vi "GetSensorType(hackversion).vi"(11 "Accessors:ID":string) -> (2 "offset":i32, 3 "SensorType":T1 items=["BumperSensor"=1, "DistanceSensor"=2, "AccelerometerSensor"=3, "Wall Sensor"=4, "Unknown"=0])   [LabVIEW 2015]
uses:
  SensorType.ctl
  <vilib>/regexp/Match Regular Expression.xnode
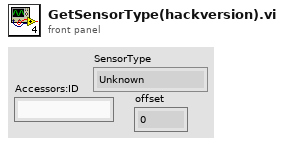
[diagram p1: front panel]
types:
  T1 = typedef "SensorType.ctl" = u16
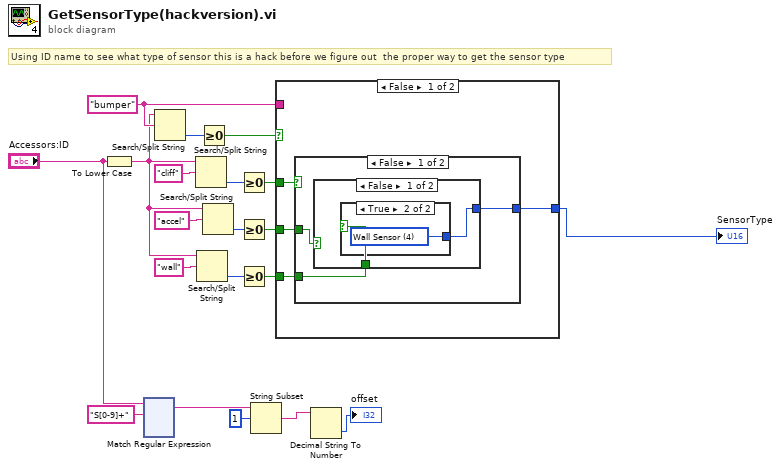
[diagram p0: block diagram]
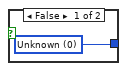
[diagram p2: hidden frame]
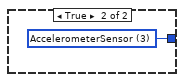
[diagram p3: hidden frame]
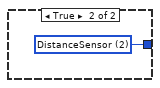
[diagram p4: hidden frame]
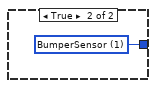
[diagram p5: hidden frame]
diagram:
  w18 = "bumper" ("search string")
  # "Using ID name to see what type of sensor this is a hack before we figure out  the proper way to get the sensor type"
  n1 = To Lower Case(string="Accessors:ID") -> (all lower case string=w9:string)
  n2 = xnode "Match Regular Expression"("input string"="Accessors:ID", "regular expression"="S[0-9]+") -> ("whole match"=w4:string)  [unwired: 4 in, 4 out]
  n3 = Search/Split String(string=w9, search string/char (-)=w18) -> (offset of match=w20:i32)  [unwired: 1 in, 2 out]
  n4 = Search/Split String(string=w9, search string/char (-)="cliff") -> (offset of match=w16:i32)  [unwired: 1 in, 2 out]
  n5 = Search/Split String(string=w9, search string/char (-)="wall") -> (offset of match=w11:i32)  [unwired: 1 in, 2 out]
  n6 = Greater Or Equal To 0?(x=w20) -> (x >= 0?=w19:bool)
  n7 = Search/Split String(string=w9, search string/char (-)="accel") -> (offset of match=w13:i32)  [unwired: 1 in, 2 out]
  n8 = Greater Or Equal To 0?(x=w16) -> (x >= 0?=w15:bool)
  n9 = Greater Or Equal To 0?(x=w13) -> (x >= 0?=w12:bool)
  n10 = Greater Or Equal To 0?(x=w11) -> (x >= 0?=w8:bool)
  n11 = String Subset(string=w4, offset (0)=1) -> (substring=w2:string)  [unwired: 1 in]
  n12 = case shown="False" w19 {
    tunnel: w18 -> [_ _]
    tunnel: [w23 w34] -> w7
    tunnel: w15 -> [w24 _]
    tunnel: w12 -> [w22 _]
    tunnel: w8 -> [w21 _]
    frame False {
      n13 = case shown="False" w24 {
        tunnel: [w27 w33] -> w23
        tunnel: w22 -> [w26 _]
        tunnel: w21 -> [w25 _]
        frame False {
          n14 = case shown="False" w26 {
            tunnel: [w28 w32] -> w27
            tunnel: w25 -> [w29 _]
            frame False {
              n15 = case shown="True" w29 {
                tunnel: [w30 w31] -> w28
                frame False {
                  w30 = T1 0 items=["BumperSensor"=1, "DistanceSensor"=2, "AccelerometerSensor"=3, "Wall Sensor"=4, "Unknown"=0] ("SensorType")
                }
                frame True {
                  w31 = T1 4 items=["BumperSensor"=1, "DistanceSensor"=2, "AccelerometerSensor"=3, "Wall Sensor"=4, "Unknown"=0] ("SensorType")
                }
              }
            }
            frame True {
              w32 = T1 3 items=["BumperSensor"=1, "DistanceSensor"=2, "AccelerometerSensor"=3, "Wall Sensor"=4, "Unknown"=0] ("SensorType")
            }
          }
        }
        frame True {
          w33 = T1 2 items=["BumperSensor"=1, "DistanceSensor"=2, "AccelerometerSensor"=3, "Wall Sensor"=4, "Unknown"=0] ("SensorType")
        }
      }
    }
    frame True {
      w34 = T1 1 items=["BumperSensor"=1, "DistanceSensor"=2, "AccelerometerSensor"=3, "Wall Sensor"=4, "Unknown"=0] ("SensorType")
    }
  }
  "SensorType" <- w7
  n16 = Decimal String To Number(string=w2) -> (number=→"offset":i32)  [unwired: 2 in, 1 out]
